vi "Configure Controller Open Response.vi"(8 "error in (no error)":errorcluster, 9 "open response":u8=128, 10 "node address (same)":u8, 11 "ProPar in":refnum<class "PL Bronkhorst ProPar.lvclass">) -> (0 "error out":errorcluster, 3 "ProPar out":refnum<class "PL Bronkhorst ProPar.lvclass">)   [LabVIEW 2015, in "PL Bronkhorst ProPar.lvclass"]
doc: "Configures controller response when starting-up from 0% of the specified <b>node</b>. Value 128 means no correction."
uses:
  PL Bronkhorst ProPar.lvclass
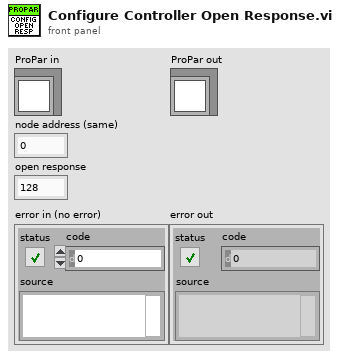
[diagram p1: front panel]
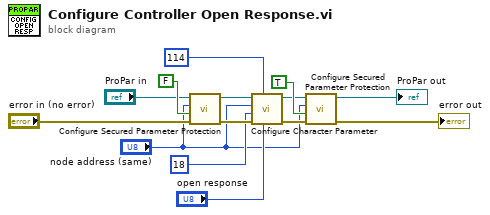
[diagram p0: block diagram]
diagram:
  n1 = call "Configure Secured Parameter Protection.vi"("enable protection"=FALSE, "node"="node address (same)", "ProPar in"="ProPar in") -> ("ProPar out"=w1:refnum<class "PL Bronkhorst ProPar.lvclass">)  [unwired: 7 in, 1 out]
  n2 = call "Configure Character Parameter.vi"("value"="open response", "process number"=u8 114, "error in (no error)"="error in (no error)", "parameter number"=u8 18 ("process number"), "node"="node address (same)", "ProPar in"=w1) -> ("error out"=w5:errorcluster, "ProPar out"=w4:refnum<class "PL Bronkhorst ProPar.lvclass">)  [unwired: 4 in]
  n3 = call "Configure Secured Parameter Protection.vi"("error in (no error)"=w5, "enable protection"=TRUE, "node"="node address (same)", "ProPar in"=w4) -> ("error out"=→"error out":errorcluster, "ProPar out"=→"ProPar out":refnum<class "PL Bronkhorst ProPar.lvclass">)  [unwired: 6 in]
